vi "Ctor.vi"(8 "error in (no error)":errorcluster) -> (0 "error out":errorcluster, 3 "WebProjectWatcher out":refnum<class "WebProjectWatcher.lvclass">)   [LabVIEW 2020, in "PicoG-Processor.lvlib" / "WebProjectWatcher.lvclass"]
uses:
  WebProjectWatcher.lvclass
  Ref Data.ctl
  Builds Callback.ctl
  WebProjectWatcher.lvclass/WebProjectWatcher.ctl
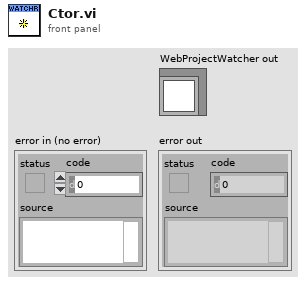
[diagram p1: front panel]
types:
  T1 = typedef "PicoG-Processor.lvlib/WebProjectWatcher.lvclass/Ref Data.ctl" = cluster{"Builds Callbacks":T2[], "Project Path":path, "Close":bool}
  T2 = typedef "PicoG-Processor.lvlib/WebProjectWatcher.lvclass/Builds Callback.ctl" = cluster{"Callback":refnum<vi>, "Owner":refnum<class>}
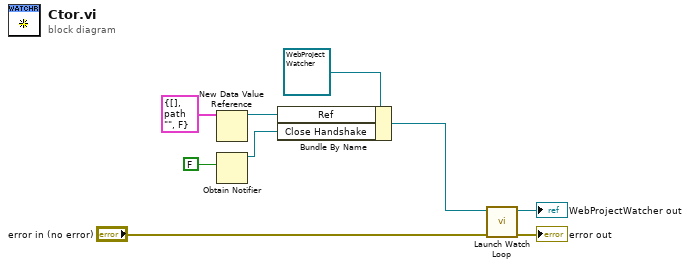
[diagram p0: block diagram]
diagram:
  n1 = New Data Value Reference(data value=T1 {"Builds Callbacks"=[], "Project Path"=path "", "Close"=FALSE} ("Ref Data")) -> (data value reference=w7:refnum<data-value>)  [unwired: 1 in, 1 out]
  n2 = Obtain Notifier(notification data type=FALSE) -> (notifier out=w1:refnum<notifier>)  [unwired: 3 in, 2 out]
  n3 = Bundle By Name(cluster=refnum<class "WebProjectWatcher.lvclass"> refnum ("WebProjectWatcher in"), "Ref"=w7, "Close Handshake"=w1) -> (w3:refnum<class "WebProjectWatcher.lvclass">)
  n4 = call "Launch Watch Loop.vi"("error in (no error)"="error in (no error)", "WebProjectWatcher in"=w3) -> ("error out"=→"error out":errorcluster, "WebProjectWatcher out"=→"WebProjectWatcher out":refnum<class "WebProjectWatcher.lvclass">)  [unwired: 8 in]
